vi "number1.vi"() -> ()   [LabVIEW 2014]
panel:
  in  "Combo Box 2":string(combo)
  in  "Combo Box":string(combo)
  out "Waveform Chart":dbl(graph)
  in  "Amp":dbl(knob) scale=0.0..10.0
  in  "freq":dbl(knob) scale=0.0..10.0
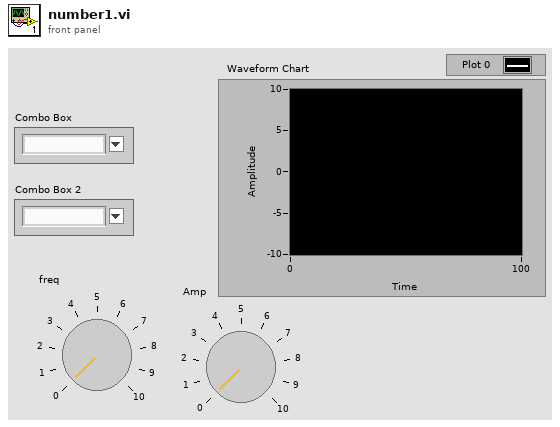
[diagram p1: front panel]
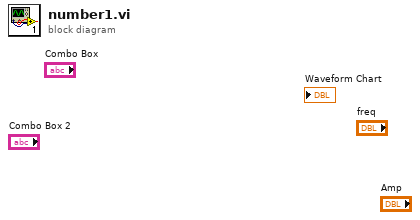
[diagram p0: block diagram]
diagram:
